vi "Splash Screen.vi"(8 "error in (no error)":errorcluster caption="에러 입력(에러 없음)") -> (0 "error out":errorcluster caption="에러 출력")   [LabVIEW 2019]
uses:
  03_Home/controller/pannelState.ctl
  <vilib>/Utility/miscctls.llb/LVPointTypeDef.ctl
  db793aa6-4e68-4d80-96e0-53e773f8ccce.vi
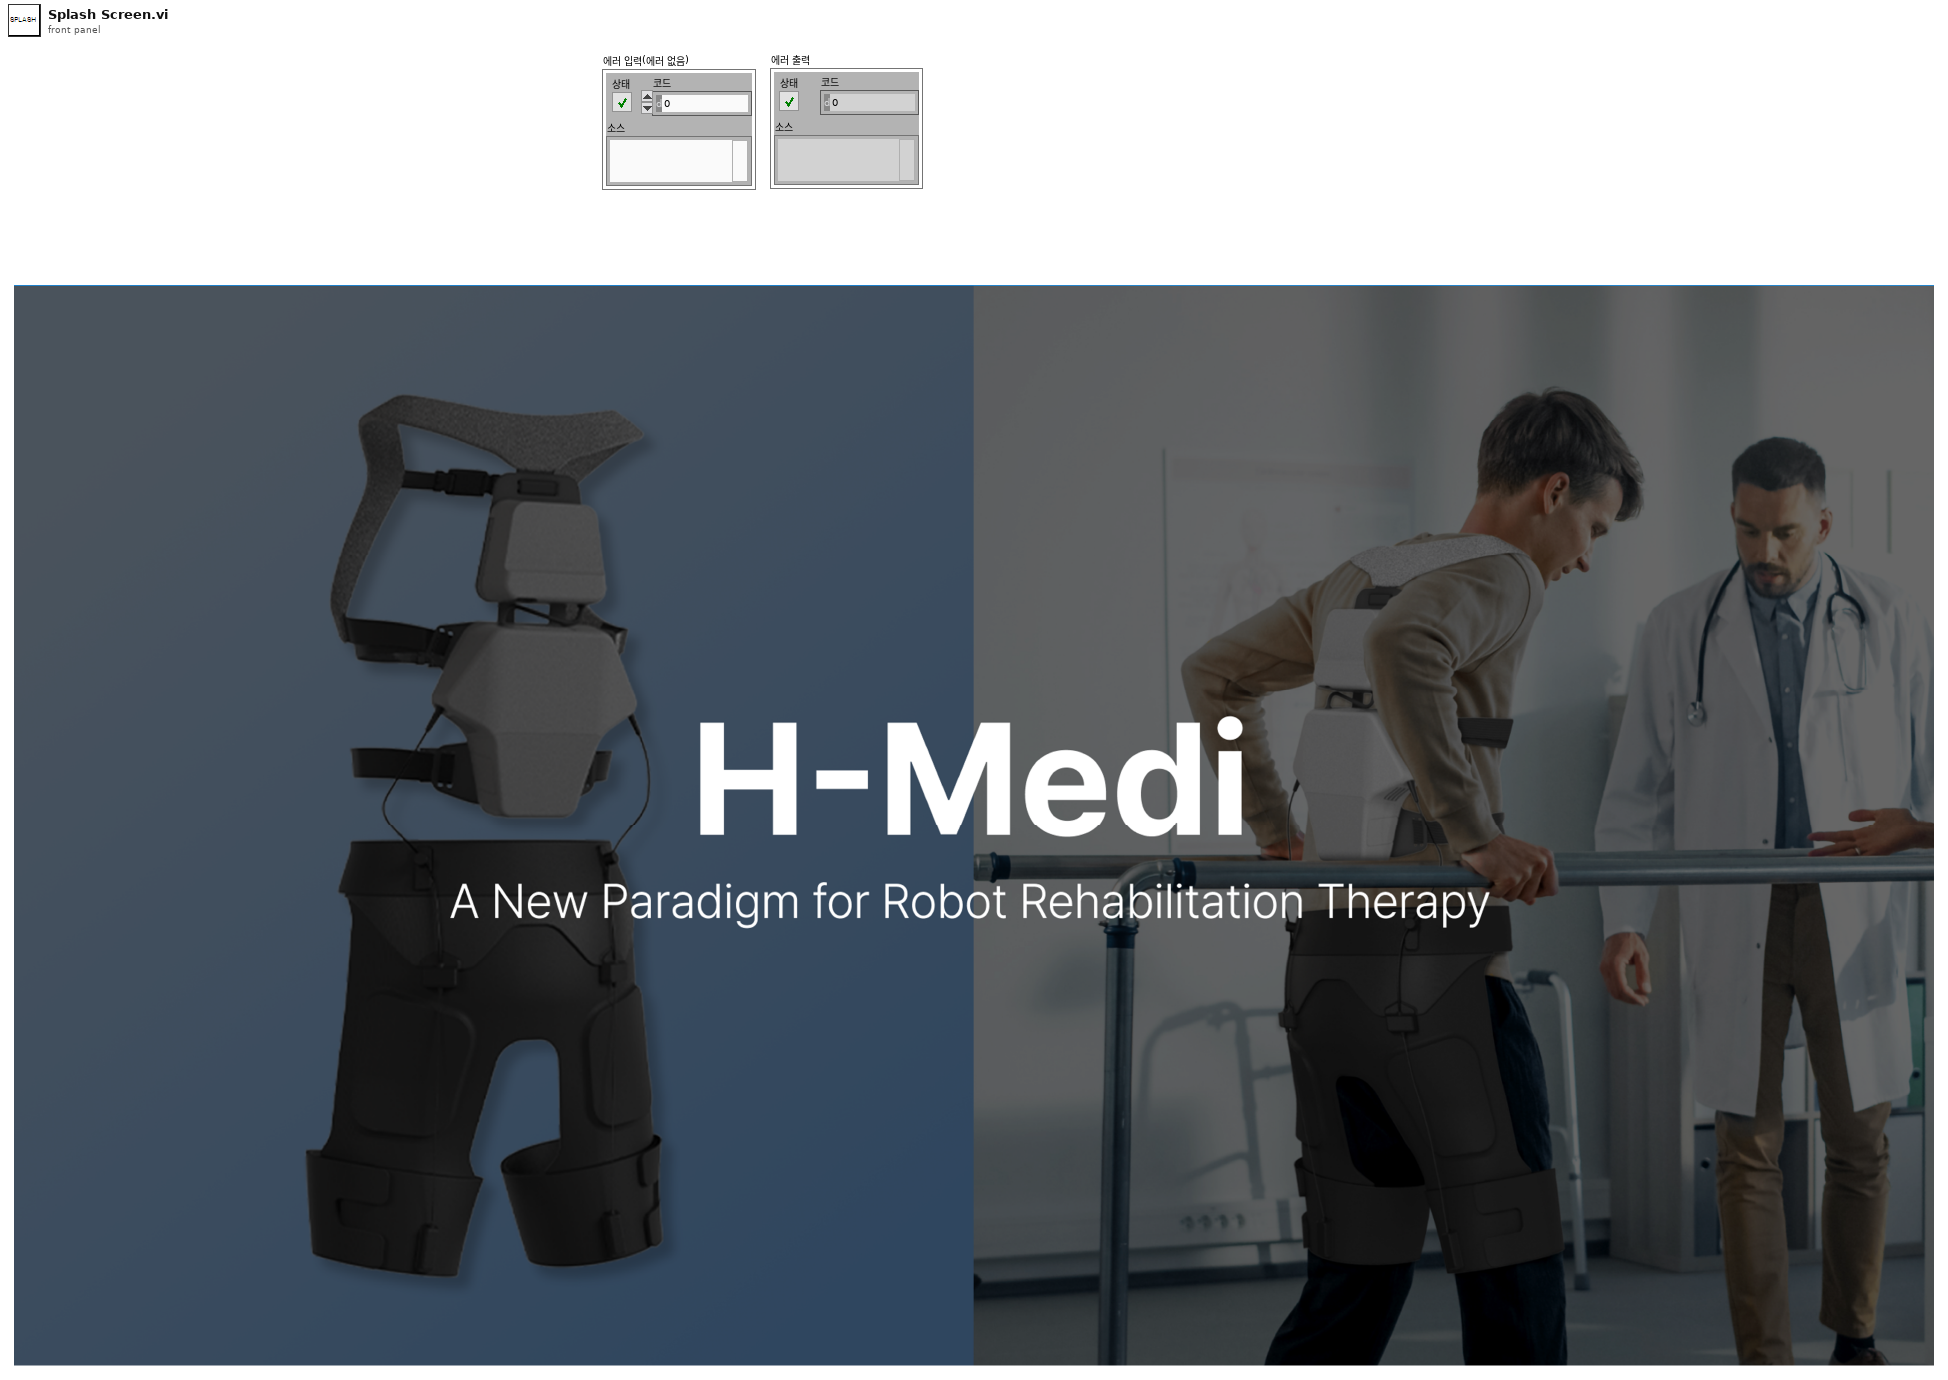
[diagram p1: front panel]
types:
  T1 = typedef "pannelState.ctl" = enum16{"Init", "LogIn", "SignUpView", "Home", "Management_patientList", "Management_patientTrashtList", "Management_patientCreate", "Management_patientUpdate", "Management_patientTraining", "Management_patientTrainingDetail", "H-MEDI PatientList", "H-MEDI HardwareCtl", "Adjust", "FineTuning", "UserList", "UserDetail", "Exit"}
  T2 = typedef "LVPointTypeDef.ctl" = cluster{"Horizontal":i16, "Vertical":i16}
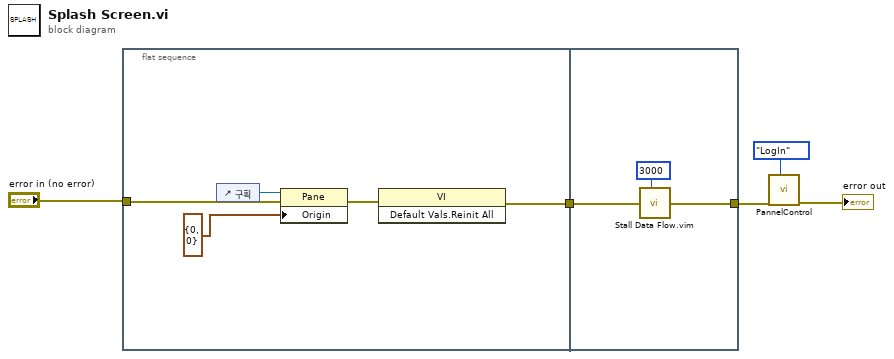
[diagram p0: block diagram]
diagram:
  n1 = flat-sequence {
    tunnel: [w7] -> w5
    tunnel: "error in (no error)" -> [w6]
    tunnel: w5 -> [w11]
    tunnel: [w13] -> w3
    frame #0 {
      n2 = control-ref of="구획"() -> (w10:refnum<vi>)
      n3 = property class="Pane"(reference=w10, error in=w6, "Origin"=T2 {"Horizontal"=0, "Vertical"=0} ("원점")) -> (error out=w9:errorcluster)  [unwired: 1 out]
      n4 = invoke class="VI" method="Default Vals.Reinit All"(error in=w9) -> (error out=w7:errorcluster)  [unwired: 2 in, 2 out]
    }
    frame #1 {
      n5 = call "Stall Data Flow.vim"("value in"=w11, "milliseconds to wait"=u32 3000) -> ("value out"=w13:errorcluster)  [unwired: 1 out]
    }
  }
  n6 = call "PannelControl.vi"("State"=pannelState."LogIn", "에러 입력(에러 없음)"=w3) -> ("error out"=→"error out":errorcluster)  [unwired: 9 in]
